vi "QFont.vi"(4 "italic":bool, 6 "weight":i32, 8 "Error In":errorcluster, 9 "pointSize":i32, 10 "family":string) -> (0 "Error Out":errorcluster, 3 "New QFont":refnum<class "QFont.lvclass">)   [LabVIEW 2014, in "QFont.lvclass"]
doc: "LabVIEW-specific documentation is not yet available. See <b>https://doc.qt.io/qt-5/qfont.html#QFont</b>"
uses:
  QFont.lvclass
  LQ Core/LQSerialData/LQSerialData.lvclass/LQSerialData.ctl
  LQ Core/LQ Core.lvlib
  LQ Core/LQSerialData/LQSerialData.lvclass
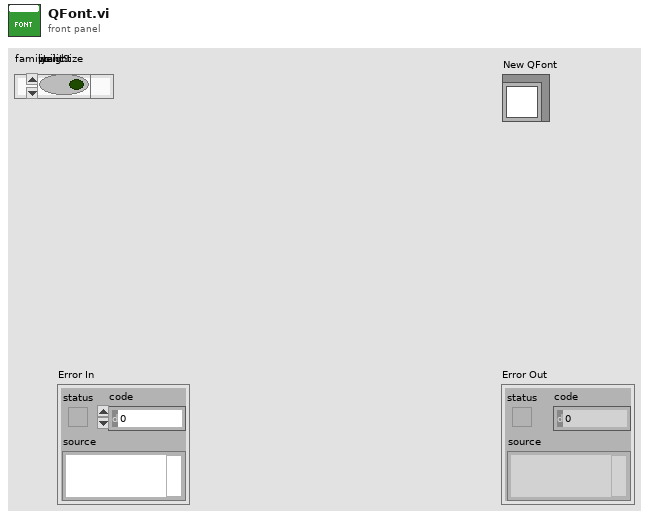
[diagram p1: front panel]
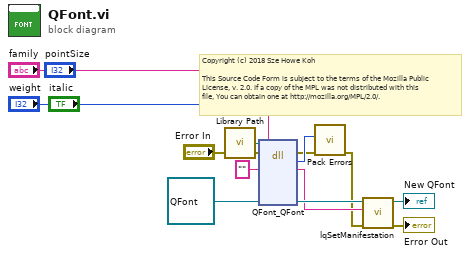
[diagram p0: block diagram]
diagram:
  # "Copyright (c) 2018 Sze Howe Koh\n\nThis Source Code Form is subject to the terms of the Mozilla Public\nLicense, v. 2.0. If a copy of the MPL was not distributed with this\nfile, You can obtain one at http://mozilla.org/MPL/2.0/."
  n1 = call "Library Path.vi"() -> ("Library Path"=w9:path)
  n2 = dll-call lib="?" fn="QFont_QFont"(path in=w9, error in="Error In", "_retVal"="", "family"="family", "pointSize"="pointSize", "weight"="weight", "italic"="italic") -> (error out=w7:errorcluster, w8:i32, "_retVal"=w10:string)  [unwired: 5 in, 1 out]
  n3 = call "Pack Errors.vi"("Error In"=w7, "Error Code"=w8) -> ("Error Out"=w6:errorcluster)  [unwired: 9 in]
  n4 = call "lqSetManifestation.vi"("Error In"=w6, "Manifestation"=w10, "LQSerialData in"=refnum<class "QFont.lvclass"> refnum ("QFont")) -> ("Error Out"=→"Error Out":errorcluster, "LQSerialData out"=→"New QFont":refnum<class "QFont.lvclass">)  [unwired: 7 in]
